vi "Query Active Channels.vi"(8 "error in (no error)":errorcluster, 11 "PicoScope 3000a in":refnum<class "PicoScope 3000a.lvclass">) -> (0 "error out":errorcluster, 2 "Active Channel(s)":T1[](array[typedef])=[enum."1"], 3 "PicoScope 3000a out":refnum<class "PicoScope 3000a.lvclass">)   [LabVIEW 2018, in "PicoScope 3000a.lvlib" / "PicoScope 3000a.lvclass"]
doc: "This methods converts the Active Channels INI configuration to:\nBoolean Array of active channels (PicoScope 3000 can have either 2 or 4 channels)\nArray of active channels in the parent class format ascend ordinally ( i.e. 1,2,3,4...), where in the case for this particular model PicoScope model A is 1 (or Channel 1), B is 2 (or Channel 2), C is 3 (or Channel 3) and D is 4 (or Channel 4)."
uses:
  PicoScope 3000a.lvclass
  LWS SLA-070/Distro/Projects/12170 Luminar LWS Base/Source/PPLs/Oscilloscope.lvlibp/Custom Controls/Analog Channels.ctl
  LWS SLA-070/Distro/Projects/12170 Luminar LWS Base/Source/PPLs/Oscilloscope.lvlibp/Oscilloscope.lvclass
  LWS SLA-070/Distro/Projects/12170 Luminar LWS Base/Source/PPLs/Oscilloscope.lvlibp
  LWS SLA-070/Distro/Projects/12170 Luminar LWS Base/Source/PPLs/Configuration.lvlibp/Configuration.lvclass
  C:/Projects/LWS SLA-070/Distro/Projects/12170 Luminar LWS Base/Source/PPLs/Oscilloscope.lvlibp/Oscilloscope.lvclass
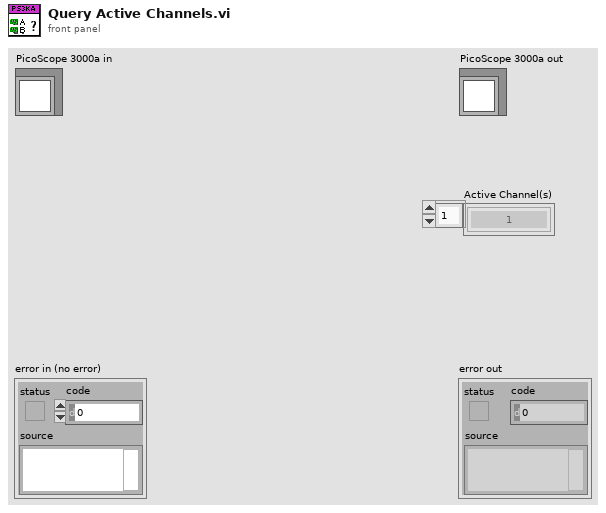
[diagram p1: front panel]
types:
  T1 = typedef "Oscilloscope.lvlibp/Analog Channels.ctl" = enum16{"1", "2", "3", "4", "5", "6", "7", "8", "9", "10", "11", "12", "13", "14", "15", "16"}
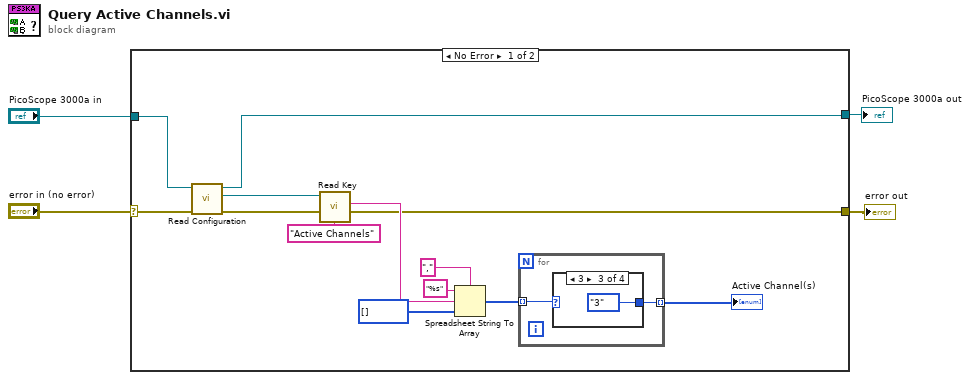
[diagram p0: block diagram]
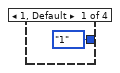
[diagram p2: hidden frame]
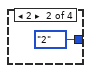
[diagram p3: hidden frame]
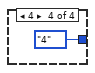
[diagram p4: hidden frame]
diagram:
  n1 = case shown="No Error" "error in (no error)" {
    selector: "error in (no error)" -> [w17 w25]
    tunnel: [w6 w25] -> w3
    tunnel: [w7 w24] -> w1
    tunnel: "PicoScope 3000a in" -> [w16 w24]
    frame No Error {
      n2 = call "Read Configuration.vi"("error in (no error)"=w17, "Oscilloscope in"=w16) -> ("error out"=w14:errorcluster, "Configuration"=w15:refnum<class "Configuration.lvclass">, "Oscilloscope out"=w7:refnum<class "PicoScope 3000a.lvclass">)  [unwired: 7 in]
      n3 = call "Read Key.vi"("Key:"="Active Channels", "error in"=w14, "Configuration in"=w15) -> ("error out"=w6:errorcluster, "Value"=w13:string)  [unwired: 6 in, 1 out]
      n4 = Spreadsheet String To Array(delimiter (Tab)=",", format string="%s", spreadsheet string=w13, array type (2D Dbl)=u32[] []) -> (array=w9:u32[])
      n5 = for {
        tunnel: w9 -> [w19] mode=indexing
        tunnel: [w18] -> w8 mode=indexing
        n6 = case shown="3" w19 {
          tunnel: [Analog_Channels."1" ("Channel") Analog_Channels."2" ("Channel") Analog_Channels."3" ("Channel") Analog_Channels."4" ("Channel")] -> w18
          frame 1, Default {
          }
          frame 2 {
          }
          frame 3 {
          }
          frame 4 {
          }
        }
      }
      "Active Channel(s)" <- w8
    }
    frame Error {
    }
  }
  "error out" <- w3
  "PicoScope 3000a out" <- w1
